vi "HAPS_LoadTable_SetBeam_Manual_Selected_Any.vi"() -> ()   [LabVIEW 2023, in "HAPS.lvlib"]
uses:
  HAPS.lvlib
  set_ele.ctl
  HAPS_SerialPort.ctl
  HAPS_MCU_ELE_Func.ctl
  <vilib>/Utility/file.llb/Read Delimited Spreadsheet (string).vi
  R_S/R_S.lvlib
panel:
  in  "offset":i32=16
  in  "H_V?":bool
  in  "IC_On/OFF":bool[][](array[boolean])=[[FALSE, FALSE, FALSE, FALSE, FALSE, FALSE, FALSE, FALSE, FALSE, FALSE, FALSE, FALSE], [FALSE, FALSE, FALSE, FALSE, FALSE, FALSE, FALSE, FALSE, FALSE, FALSE, FALSE, FALSE], [FALSE, FALSE, FALSE, FALSE, FALSE, FALSE, FALSE, FALSE, FALSE, FALSE, FALSE, FALSE]]
  in  "ele_gain?":i32=35
  in  "sys reboot?":bool=TRUE
  in  "VISA resource name":refnum<visa-resource-name>="COM1"
  in  "file path":path=path "D:/_Project/_Code/LabVIEW/_CLC_Gen4/CLC_LV2023/CLC_Cali/Log/HAPS/Preset.csv"
  out "error IO":errorcluster
  out "Err_code":i32
  out "status":bool
  in  "offset?":bool
  in  "simu.?":bool
  in  "set_ele":T1={"ch"=0, "chain_id"=0, "group"=0, "array_id"=0, "ele_phase"=0, "ele_gain"=35, "com_gain"=17, "pd_range"=0}
  out "ele phase":i32
  out "ele gain":i32
  out "channel":i32
  out "chain ID":i32
  out "group":i32
  out "array id":i32
  # "HAPS 24x24 Setting Manual In-Phase : \n                                                           Any BFIC"
  # "Tx:35\nRx:22"
  # "0"
  # "5"
  # "6"
  # "11"
  # "Group_0"
  # "Group_1"
  # "Group_2"
  # "Not using!!!!!!!!!!!!!!!!!!!!!!!!!!!!!!!!!!!!!!!!"
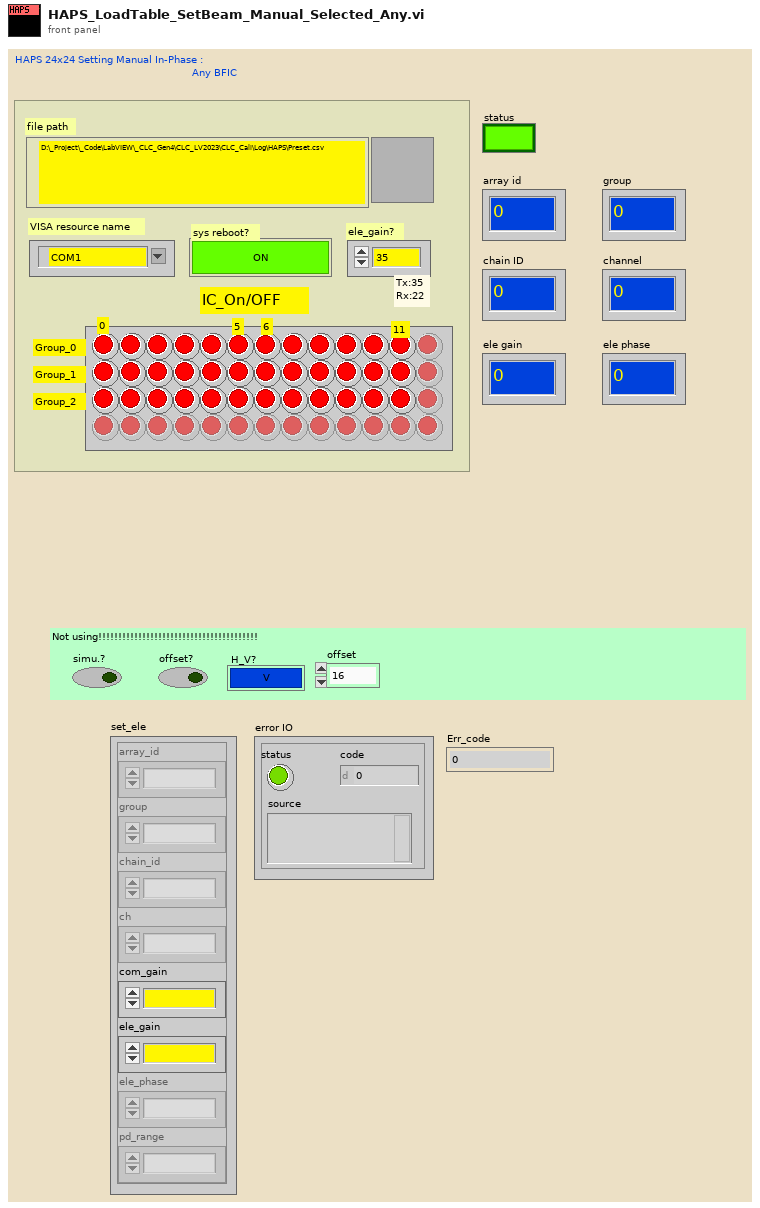
[diagram p1: front panel]
types:
  T1 = typedef "HAPS.lvlib/set_ele.ctl" = cluster{"ch":i32, "chain_id":i32, "group":i32, "array_id":i32, "ele_phase":i32, "ele_gain":i32, "com_gain":i32, "pd_range":i32}
  T2 = typedef "HAPS.lvlib/HAPS_SerialPort.ctl" = enum16{"Init", "Close", "CMD", "Flush"}
  T3 = typedef "HAPS.lvlib/HAPS_MCU_ELE_Func.ctl" = enum16{"array_init", "set_com_gain", "set_ch_gain_phase", "set_pd_range", "get_preamp_temp", "get_bfic_temp", "get_tx_pd", "ch_on", "ch_on_2", "ch_ctrl_all", "array_ctrl_src"}
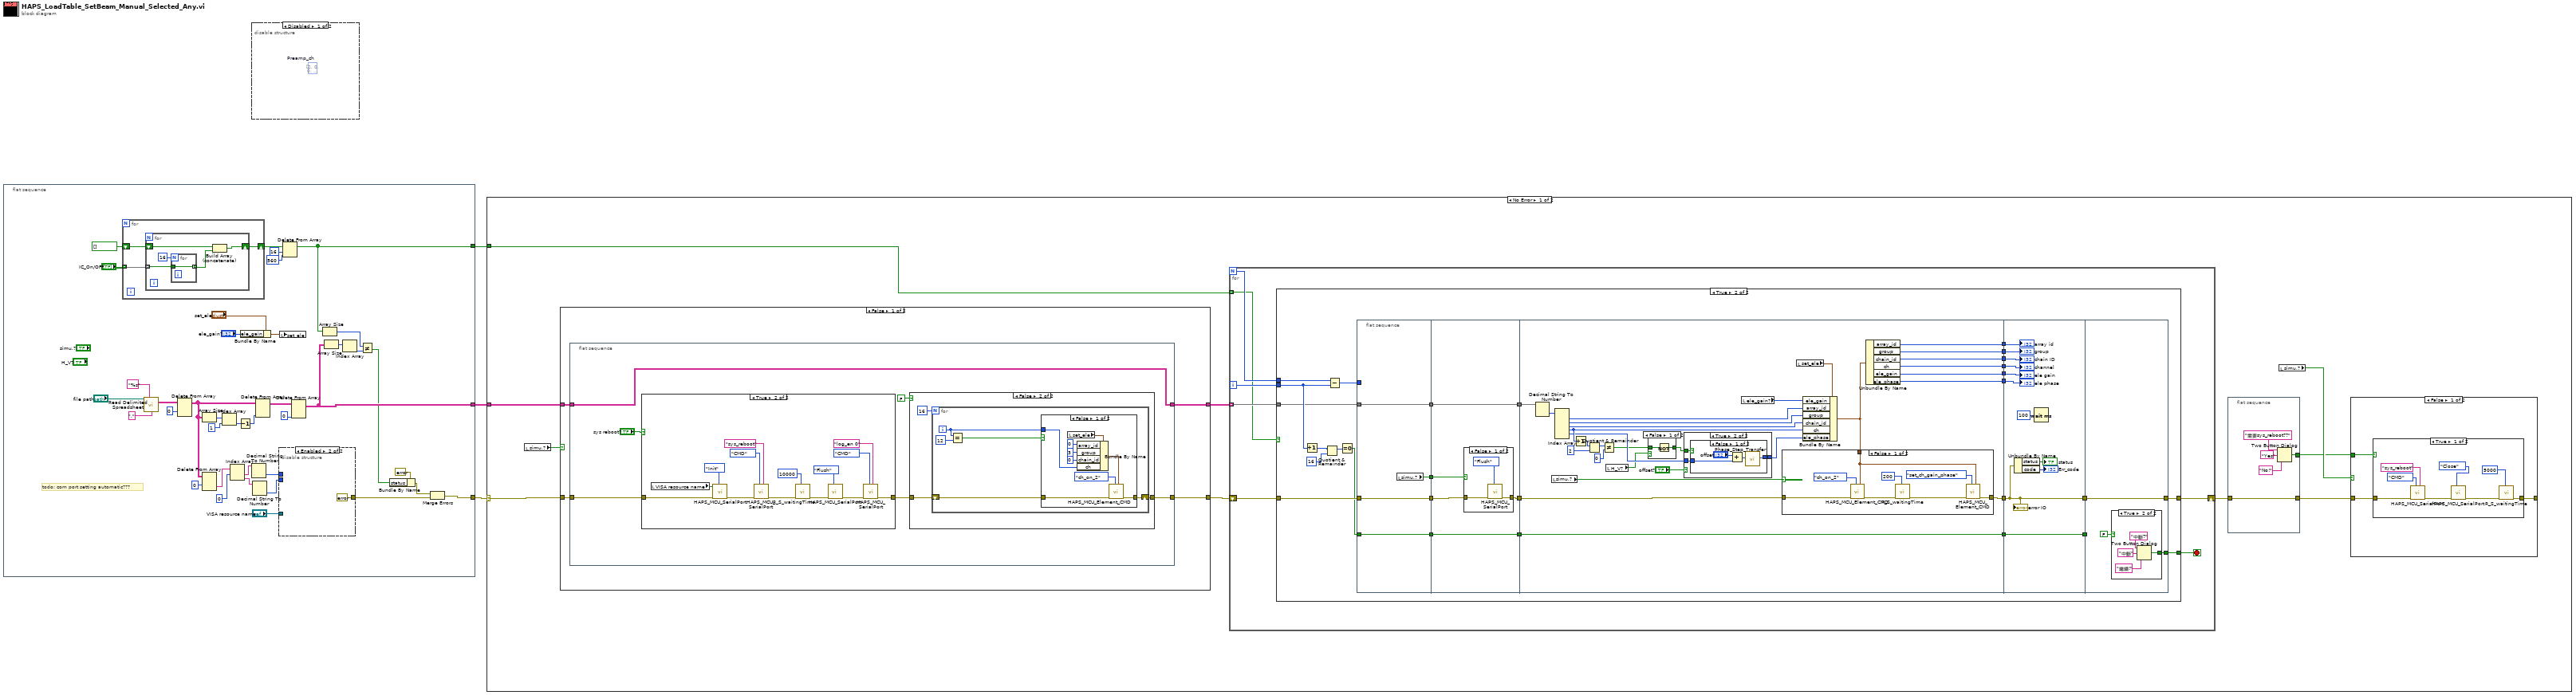
[diagram p0: block diagram]
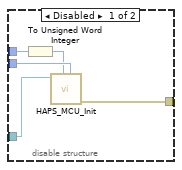
[diagram p2: hidden frame]
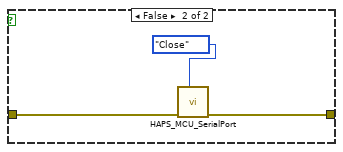
[diagram p4: hidden frame]
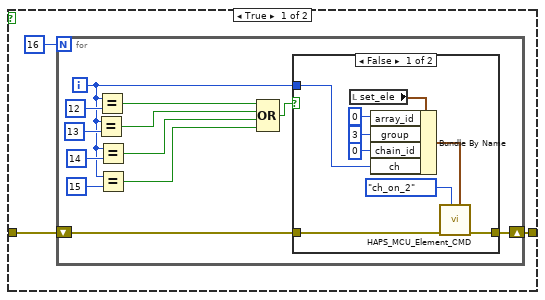
[diagram p6: hidden frame]
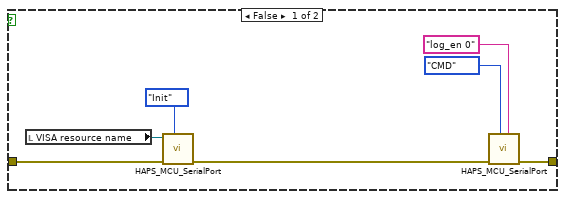
[diagram p9: hidden frame]
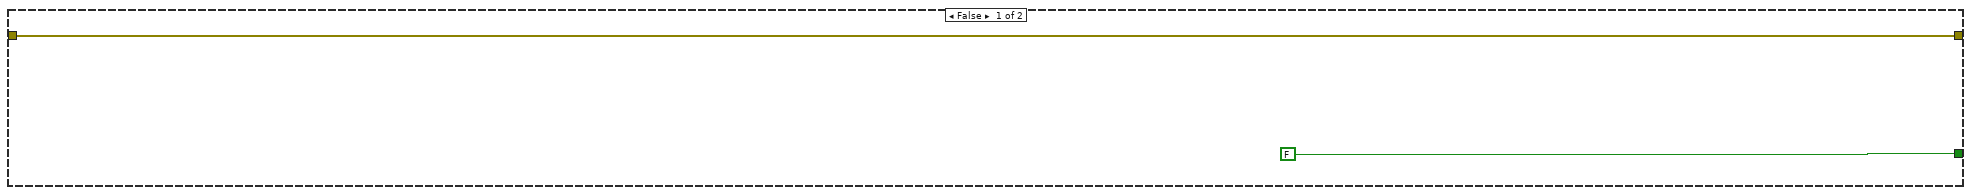
[diagram p11: hidden frame]
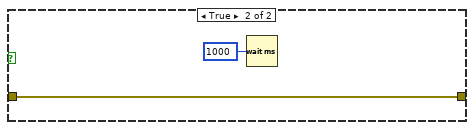
[diagram p16: hidden frame]
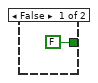
[diagram p17: hidden frame]
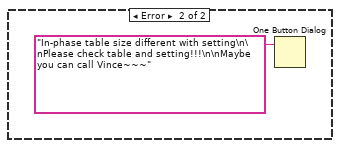
[diagram p18: hidden frame]
diagram:
  n1 = flat-sequence {
    tunnel: [w7] -> w3
    tunnel: [w11] -> w2
    tunnel: [w12] -> w1
    frame #0 {
      # "todo: com port setting automatic???"
      n2 = for {
        tunnel: "IC_On/OFF" -> [w44] mode=indexing
        shift-right: [w42] -> w17
        shift-left: bool[] [] -> [w43]
        n3 = for {
          tunnel: w44 -> [w48] mode=indexing
          shift-right: [w45] -> w42
          shift-left: w43 -> [w46]
          n4 = for {
            N: 16 -> [_]
            tunnel: w48 -> [w50]
            tunnel: [w50] -> w47 mode=indexing
          }
          n5 = Build Array (concatenate)(w46, w47) -> (w45:bool[])
        }
      }
      n6 = call-poly <vilib>:"Read Delimited Spreadsheet.vi"("file path (dialog if empty)"="file path", "format (%s)"="%s" ("format (%.3f)"), "delimiter (\\t)"="," ("delimiter (\\t)")) -> ("all rows"=w39:string[][])  [unwired: 7 in, 5 out]
      n7 = Delete From Array(array=w39, index (row)=0) -> (array with subset deleted=w29:string[][])  [unwired: 2 in, 1 out]
      n8 = Array Size(array=w29) -> (size(s)=w37:i32[])
      n9 = Delete From Array(array=w29, index (row)=0) -> (deleted portion=w28:string[])  [unwired: 2 in, 1 out]
      n10 = Index Array(array=w37, index=1) -> (element=w34:i32)
      n11 = Index Array(array=w28, index #1=0 ("index")) -> (element #1=w27:string, element #2=w26:string)  [unwired: 1 in]
      n12 = Decrement(x=w34) -> (x-1=w36:i32)
      n13 = Bundle By Name(cluster="set_ele", "ele_gain"="ele_gain?") -> (w18:T1)
      n14 = Decimal String To Number(string=w27) -> (number=w23:i32)  [unwired: 2 in, 1 out]
      n15 = Decimal String To Number(string=w26) -> (number=w22:i32)  [unwired: 2 in, 1 out]
      n16 = Delete From Array(array=w29, index (col)=w36) -> (array with subset deleted=w32:string[][])  [unwired: 2 in, 1 out]
      n17 = disable-structure shown="Enabled" {
        disable-tunnel: [w55 errorcluster {"status"=FALSE, "code"=0, "source"=""} ("error out")] -> w33
        disable-tunnel: w23 -> [w54 _]
        disable-tunnel: w22 -> [w53 _]
        disable-tunnel: "VISA resource name" -> [w52 _]
        frame Disabled {
          n18 = To Unsigned Word Integer(number=w54) -> (unsigned 16bit integer=w51:u16)
          n19 = call "HAPS_MCU_Init.vi"("array_id"=w53, "Tx/Rx"=w51, "VISA resource name"=w52) -> ("error out"=w55:errorcluster)  [unwired: 8 in]
        }
        frame Enabled {
        }
      }
      n20 = local write "set_ele"(w18) -> ()
      n21 = Delete From Array(array=w17, length=16, index=560) -> (array with subset deleted=w12:bool[])  [unwired: 1 out]
      n22 = Delete From Array(array=w32, index (col)=0 ("index (row)")) -> (array with subset deleted=w11:string[][])  [unwired: 2 in, 1 out]
      n23 = Array Size(array=w12) -> (size(s)=w9:i32)
      n24 = Array Size(array=w11) -> (size(s)=w10:i32[])
      n25 = Index Array(array=w10) -> (element=w8:i32)  [unwired: 1 in]
      n26 = Not Equal?(x=w9, y=w8) -> (x != y?=w5:bool)
      n27 = Bundle By Name(cluster=errorcluster {"status"=FALSE, "code"=0, "source"=""} ("error out"), "status"=w5) -> (w4:errorcluster)
      n28 = Merge Errors(w4, w33) -> (w7:errorcluster)
    }
  }
  n29 = disable-structure shown="Disabled" {
    frame Disabled {
      (unwired) i32[][] [[2, 0, 0, 8, 8, 10, 11, 9, 9, 1, 1, 3], [3, 1, 1, 9, 9, 11, 13, 15, 15, 7, 7, 5], [5, 7, 7, 15, 15, 13, 14, 14, 6, 6, 4, 12]]  # Preamp_ch
    }
    frame Enabled {
    }
  }
  n30 = case shown="No Error" w3 {
    selector: w3 -> [w64 _]
    tunnel: w2 -> [w66 _]
    tunnel: w1 -> [w60 _]
    frame No Error {
      n31 = local read "simu.?"() -> (w62:bool)
      n32 = case shown="False" w62 {
        tunnel: w66 -> [w90 w162]
        tunnel: [w89 w162] -> w65
        tunnel: w64 -> [w88 w161]
        tunnel: [w87 w161] -> w63
        frame False {
          n33 = flat-sequence {
            tunnel: w90 -> [w96]
            tunnel: [w96] -> w89
            tunnel: w88 -> [w94]
            tunnel: [w95] -> w87
            frame #0 {
              n34 = case shown="True" "sys reboot?" {
                tunnel: w94 -> [w144 w158]
                tunnel: [w142 w156] -> w93
                frame False {
                  n35 = local read "VISA resource name"() -> (w140:refnum<visa-resource-name>)
                  n36 = call "HAPS_MCU_SerialPort.vi"("HAPS_SerialPort_Func"=HAPS_SerialPort."Init", "error in"=w144, "VISA resource name"=w140) -> ("error out"=w141:errorcluster)  [unwired: 6 in, 2 out]
                  n37 = call "HAPS_MCU_SerialPort.vi"("Command"="log_en 0", "HAPS_SerialPort_Func"=enum16{"Init", "Close", "CMD"}."CMD" ("HAPS_SerialPort"), "error in"=w141) -> ("error out"=w142:errorcluster)  [unwired: 6 in, 2 out]
                }
                frame True {
                  n38 = local read "VISA resource name"() -> (w147:refnum<visa-resource-name>)
                  n39 = call "HAPS_MCU_SerialPort.vi"("HAPS_SerialPort_Func"=HAPS_SerialPort."Init", "error in"=w158, "VISA resource name"=w147) -> ("error out"=w153:errorcluster)  [unwired: 6 in, 2 out]
                  n40 = call "HAPS_MCU_SerialPort.vi"("Command"="sys_reboot", "HAPS_SerialPort_Func"=enum16{"Init", "Close", "CMD"}."CMD" ("HAPS_SerialPort"), "error in"=w153) -> ("error out"=w152:errorcluster)  [unwired: 6 in, 2 out]
                  n41 = call "R_S_waitingTime.vi"("Waiting Time(ms)"=u32 10000, "error in"=w152) -> ("error out"=w150:errorcluster)  [unwired: 9 in]
                  n42 = call "HAPS_MCU_SerialPort.vi"("HAPS_SerialPort_Func"=HAPS_SerialPort."Flush", "error in"=w150) -> ("error out"=w148:errorcluster)  [unwired: 7 in, 2 out]
                  n43 = call "HAPS_MCU_SerialPort.vi"("Command"="log_en 0", "HAPS_SerialPort_Func"=enum16{"Init", "Close", "CMD"}."CMD" ("HAPS_SerialPort"), "error in"=w148) -> ("error out"=w156:errorcluster)  [unwired: 6 in, 2 out]
                }
              }
              n44 = case shown="False" FALSE {
                tunnel: [w98 w123] -> w95
                tunnel: w93 -> [w97 w122]
                frame True {
                  n45 = for {
                    N: 16 -> [_]
                    shift-right: [w110] -> w98
                    shift-left: w97 -> [w111]
                    i -> [w101]
                    n46 = Equal?(x=w101, y=13) -> (x = y?=w105:bool)
                    n47 = Equal?(x=w101, y=12) -> (x = y?=w109:bool)
                    n48 = Equal?(x=w101, y=14) -> (x = y?=w103:bool)
                    n49 = Equal?(x=w101, y=15) -> (x = y?=w100:bool)
                    n50 = Compound Arithmetic op=OR(w109, w105, w103, w100) -> (w106:bool)
                    n51 = case shown="False" w106 {
                      tunnel: w111 -> [w114 w121]
                      tunnel: [w113 w121] -> w110
                      tunnel: w101 -> [w112 _]
                      frame False {
                        n52 = local read "set_ele"() -> (w116:T1)
                        n53 = Bundle By Name(cluster=w116, "array_id"=0, "group"=3, "chain_id"=0, "ch"=w112) -> (w117:T1)
                        n54 = call "HAPS_MCU_Element_CMD.vi"("set_ele"=w117, "HAPS_MCU_ELE_Func."=HAPS_MCU_ELE_Func."ch_on_2", "error in"=w114) -> ("error out"=w113:errorcluster)  [unwired: 7 in, 1 out]
                      }
                      frame True {
                      }
                    }
                  }
                }
                frame False {
                  n55 = for {
                    N: 16 -> [_]
                    shift-right: [w128] -> w123
                    shift-left: w122 -> [w129]
                    i -> [w126]
                    n56 = Equal?(x=w126, y=12) -> (x = y?=w125:bool)
                    n57 = case shown="False" w125 {
                      tunnel: w129 -> [w132 w139]
                      tunnel: [w131 w139] -> w128
                      tunnel: w126 -> [w130 _]
                      frame False {
                        n58 = local read "set_ele"() -> (w134:T1)
                        n59 = Bundle By Name(cluster=w134, "array_id"=0, "group"=3, "chain_id"=0, "ch"=w130) -> (w135:T1)
                        n60 = call "HAPS_MCU_Element_CMD.vi"("set_ele"=w135, "HAPS_MCU_ELE_Func."=HAPS_MCU_ELE_Func."ch_on_2", "error in"=w132) -> ("error out"=w131:errorcluster)  [unwired: 7 in, 1 out]
                      }
                      frame True {
                      }
                    }
                  }
                }
              }
            }
          }
        }
        frame True {
        }
      }
      n61 = for {
        N -> [w167]
        tunnel: w65 -> [w165] mode=indexing
        shift-right: [w169] -> w59
        shift-left: w63 -> [w168]
        tunnel: w60 -> [w163] mode=indexing
        i -> [w166]
        stop <- w164 stop-if-true
        n62 = case shown="True" w163 {
          tunnel: [w170 w183] -> w169
          tunnel: w168 -> [w170 w182]
          tunnel: w167 -> [_ w181]
          tunnel: w166 -> [_ w180]
          tunnel: w165 -> [_ w179]
          tunnel: [FALSE ("T button?") w173] -> w164
          frame False {
          }
          frame True {
            n63 = Increment(x=w180) -> (x+1=w177:i32)
            n64 = Quotient & Remainder(x=w177, y=16) -> (x-y*floor(x/y)=w175:i32)  [unwired: 1 out]
            n65 = Subtract(x=w181, y=w180) -> (x-y=w178:i32)
            n66 = Equal To 0?(x=w175) -> (x = 0?=w174:bool)
            n67 = flat-sequence {
              tunnel: w178 -> [_]
              tunnel: w182 -> [w202]
              tunnel: w179 -> [w203]
              tunnel: [w203] -> w199
              tunnel: [w202] -> w198
              tunnel: w174 -> [w201]
              tunnel: [w201] -> w197
              tunnel: [w200] -> w172
              tunnel: [w208] -> w196
              tunnel: [w207] -> w195
              tunnel: w199 -> [w208]
              tunnel: w198 -> [w206]
              tunnel: w197 -> [w205]
              tunnel: [w205] -> w194
              tunnel: w172 -> [w204]
              tunnel: w196 -> [w241]
              tunnel: w195 -> [w239]
              tunnel: [w227] -> w193
              tunnel: [w237] -> w192
              tunnel: [w236] -> w191
              tunnel: [w235] -> w190
              tunnel: [w234] -> w189
              tunnel: [w233] -> w188
              tunnel: [w232] -> w187
              tunnel: w194 -> [w228]
              tunnel: [w228] -> w186
              tunnel: w193 -> [w266]
              tunnel: w192 -> [w274]
              tunnel: w191 -> [w273]
              tunnel: w190 -> [w272]
              tunnel: w189 -> [w271]
              tunnel: w188 -> [w270]
              tunnel: w187 -> [w269]
              tunnel: [w266] -> w185
              tunnel: w186 -> [w267]
              tunnel: [w267] -> w184
              tunnel: w185 -> [w277]
              tunnel: w184 -> [_]
              tunnel: [w277] -> w183
              tunnel: [w276] -> w173
              frame #0 {
                n68 = local read "simu.?"() -> (w200:bool)
              }
              frame #1 {
                n69 = case shown="False" w204 {
                  tunnel: [w211 w212] -> w207
                  tunnel: w206 -> [w210 w212]
                  frame False {
                    n70 = call "HAPS_MCU_SerialPort.vi"("HAPS_SerialPort_Func"=HAPS_SerialPort."Flush", "error in"=w210) -> ("error out"=w211:errorcluster)  [unwired: 7 in, 2 out]
                  }
                  frame True {
                  }
                }
              }
              frame #2 {
                n71 = Decimal String To Number(string=w241) -> (number=w240:i32[])  [unwired: 2 in, 1 out]
                n72 = local read "simu.?"() -> (w226:bool)
                n73 = Index Array(array=w240) -> (element #1=w238:i32, element #2=w231:i32, element #3=w230:i32, element #4=w224:i32, element #5=w220:i32)  [unwired: 6 in, 1 out]
                n74 = Increment(x=w224) -> (x+1=w217:i32)
                n75 = Quotient & Remainder(x=w217, y=2) -> (x-y*floor(x/y)=w222:i32)  [unwired: 1 out]
                n76 = Not Equal?(x=w222, y=0) -> (x != y?=w214:bool)
                n77 = local read "H_V?"() -> (w215:bool)
                n78 = case shown="False" w215 {
                  tunnel: w214 -> [w243 w244]
                  tunnel: [w242 w244] -> w213
                  frame False {
                    n79 = Not(x=w243) -> (.not. x?=w242:bool)
                  }
                  frame True {
                  }
                }
                n80 = case shown="True" "offset?" {
                  tunnel: w220 -> [w245 w248]
                  tunnel: w213 -> [_ w247]
                  tunnel: [w245 w246] -> w219
                  frame False {
                  }
                  frame True {
                    n81 = case shown="False" w247 {
                      tunnel: w248 -> [w252 w253]
                      tunnel: [w249 w253] -> w246
                      frame False {
                        n82 = Add(x="offset", y=w252) -> (x+y=w250:i32)
                        n83 = call "Phase_Step_Transfer.vi"("Input_Phase_Step"=w250) -> ("Output_Phase_Step"=w249:i32)  [unwired: 10 in]
                      }
                      frame True {
                      }
                    }
                  }
                }
                n84 = local read "ele_gain?"() -> (w216:i32)
                n85 = local read "set_ele"() -> (w229:T1)
                n86 = Bundle By Name(cluster=w229, "ele_gain"=w216, "array_id"=w238, "group"=w231, "chain_id"=w230, "ch"=w224, "ele_phase"=w219) -> (w225:T1)
                n87 = case shown="False" w226 {
                  tunnel: w239 -> [w261 w263]
                  tunnel: w225 -> [w260 _]
                  tunnel: [w259 w263] -> w227
                  frame False {
                    n88 = call "HAPS_MCU_Element_CMD.vi"("set_ele"=w260, "HAPS_MCU_ELE_Func."=HAPS_MCU_ELE_Func."ch_on_2", "error in"=w261) -> ("error out"=w255:errorcluster)  [unwired: 7 in, 1 out]
                    n89 = call "R_S_waitingTime.vi"("Waiting Time(ms)"=u32 200, "error in"=w255) -> ("error out"=w254:errorcluster)  [unwired: 9 in]
                    n90 = call "HAPS_MCU_Element_CMD.vi"("set_ele"=w260, "HAPS_MCU_ELE_Func."=HAPS_MCU_ELE_Func."set_ch_gain_phase", "error in"=w254) -> ("error out"=w259:errorcluster)  [unwired: 7 in, 1 out]
                  }
                  frame True {
                    n91 = Wait (ms)(milliseconds to wait=u32 1000) -> ()  [unwired: 1 out]
                  }
                }
                n92 = Unbundle By Name(w225) -> ("array_id"=w237:i32, "group"=w236:i32, "chain_id"=w235:i32, "ch"=w234:i32, "ele_gain"=w233:i32, "ele_phase"=w232:i32)
              }
              frame #3 {
                n93 = Unbundle By Name(w266) -> ("status"=→"status":bool, "code"=→"Err_code":i32)
                n94 = Wait (ms)(milliseconds to wait=u32 100) -> ()  [unwired: 1 out]
                "group" <- w273
                "chain ID" <- w272
                "channel" <- w271
                "ele gain" <- w270
                "ele phase" <- w269
                "array id" <- w274
                "error IO" <- w266
              }
              frame #4 {
                n95 = case shown="True" FALSE {
                  tunnel: [FALSE ("T button?") w281] -> w276
                  frame False {
                  }
                  frame True {
                    n96 = Two Button Dialog(message="中斷?", 1:"繼續!" ("F button name (\"Cancel\")"), 2:"中斷" ("T button name (\"OK\")")) -> (T button?=w281:bool)
                  }
                }
              }
            }
          }
        }
      }
      n97 = flat-sequence {
        tunnel: w59 -> [w71]
        tunnel: [w71] -> w58
        tunnel: [w67] -> w57
        frame #0 {
          n98 = Two Button Dialog(message="需要sys_reboot??", 1:"No!" ("F button name (\"Cancel\")"), 2:"Yes" ("T button name (\"OK\")")) -> (T button?=w67:bool)
        }
      }
      n99 = local read "simu.?"() -> (w61:bool)
      n100 = case shown="False" w61 {
        tunnel: [w73 w86] -> _
        tunnel: w58 -> [w74 w86]
        tunnel: w57 -> [w72 _]
        frame False {
          n101 = case shown="True" w72 {
            tunnel: w74 -> [w82 w84]
            tunnel: [w75 w83] -> w73
            frame True {
              n102 = call "HAPS_MCU_SerialPort.vi"("Command"="sys_reboot", "HAPS_SerialPort_Func"=enum16{"Init", "Close", "CMD"}."CMD" ("HAPS_SerialPort"), "error in"=w82) -> ("error out"=w78:errorcluster)  [unwired: 6 in, 2 out]
              n103 = call "HAPS_MCU_SerialPort.vi"("HAPS_SerialPort_Func"=HAPS_SerialPort."Close", "error in"=w78) -> ("error out"=w76:errorcluster)  [unwired: 7 in, 2 out]
              n104 = call "R_S_waitingTime.vi"("Waiting Time(ms)"=u32 5000, "error in"=w76) -> ("error out"=w75:errorcluster)  [unwired: 9 in]
            }
            frame False {
              n105 = call "HAPS_MCU_SerialPort.vi"("HAPS_SerialPort_Func"=HAPS_SerialPort."Close", "error in"=w84) -> ("error out"=w83:errorcluster)  [unwired: 7 in, 2 out]
            }
          }
        }
        frame True {
        }
      }
    }
    frame Error {
      n106 = One Button Dialog(message="In-phase table size different with setting\n\nPlease check table and setting!!!\n\nMaybe you can call Vince~~~") -> ()  [unwired: 1 in, 1 out]
    }
  }
